vi "Calibrate IQ.vi"(6 "Stop Frequency (100 kHz)":dbl=100000.0, 8 "error in (no error)":errorcluster, 9 "Start Frequency (100 kHz)":dbl=100000.0, 10 "Calibration Type (0: User)":u16(ring) items=["User", "Revert to default", "Full"], 11 "VISA resource name":refnum<visa-resource-name>) -> (0 "error out":errorcluster, 3 "VISA resource name out":refnum<visa-resource-name>)   [LabVIEW 2012, in "Agilent PSG MXG Series.lvlib"]
doc: "Configures the calibration type and range for an I/Q calibration.\n\n<B>Notes:</B>\n(1) This VI is valid only in E8267C, E8267D, N5162A, N5182A, N5172B, N5182B.\n\n(2) For N5162A and N5182A, this VI is valid only when the instrument installs <B>Option 651</B> or <B>Option 652</B> or <B>Option 654</B> (Internal baseband generator).\n\n(3) For N5172B, this VI is valid only when the instrument installs <B>Option 653</B> or <B>Option 655</B>.\n\n(4) For N5182B, this VI is valid only when the instrument installs <B>Option 656</B> or <B>Option 657</B>."
uses:
  <instrlib>/Agilent PSG MXG Series/Agilent PSG MXG Series.lvlib
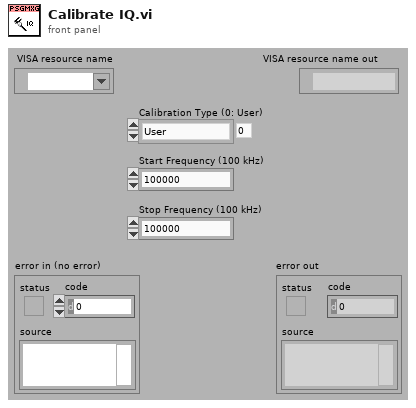
[diagram p1: front panel]
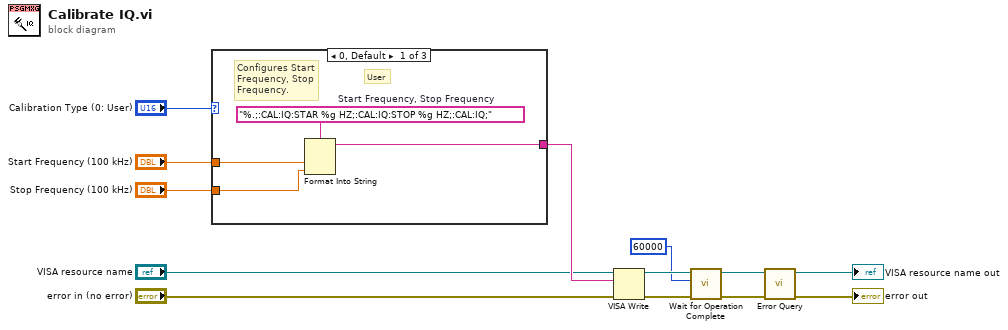
[diagram p0: block diagram]
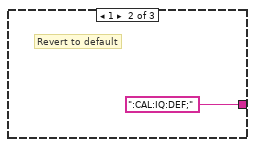
[diagram p2: hidden frame]
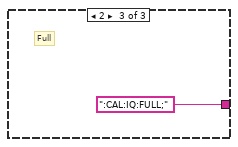
[diagram p3: hidden frame]
diagram:
  n1 = case shown="0, Default" "Calibration Type (0: User)" {
    tunnel: "Start Frequency (100 kHz)" -> [w16 _ _]
    tunnel: "Stop Frequency (100 kHz)" -> [w15 _ _]
    tunnel: [w14 ":CAL:IQ:DEF;" ":CAL:IQ:FULL;"] -> w10
    frame 0, Default {
      w17 = "%.;:CAL:IQ:STAR %g HZ;:CAL:IQ:STOP %g HZ;:CAL:IQ;"  # Start Frequency, Stop Frequency
      # "Configures Start\nFrequency, Stop\nFrequency."
      # "User"
      n2 = Format Into String(format string=w17, w16, w15) -> (resulting string=w14:string)  [unwired: 2 in, 1 out]
    }
    frame 1 {
      # "Revert to default"
    }
    frame 2 {
      # "Full"
    }
  }
  n3 = VISA Write(VISA resource name="VISA resource name", write buffer=w10, error in (no error)="error in (no error)") -> (VISA resource name out=w9:refnum<visa-resource-name>, error out=w8:errorcluster)  [unwired: 1 out]
  n4 = call <instrlib>:"Wait for Operation Complete.vi"("error in (no error)"=w8, "Maximum Time (10000 ms)"=60000, "VISA resource name"=w9) -> ("error out"=w5:errorcluster, "VISA resource name out"=w6:refnum<visa-resource-name>)  [unwired: 7 out]
  n5 = call <instrlib>:"Error Query.vi"("error in (no error)"=w5, "VISA resource name"=w6) -> ("error out"=→"error out":errorcluster, "VISA resource name out"=→"VISA resource name out":refnum<visa-resource-name>)  [unwired: 8 out]
